vi "getInstanceMsg.vi"(8 "error in (no error)":errorcluster, 11 "tcpServer in":refnum<class "TcpServer.lvclass">) -> (0 "error out":errorcluster, 1 "MsgWrite":refnum<user-event>, 2 "MsgRead":refnum<user-event>, 3 "tcpServer out":refnum<class "TcpServer.lvclass">)   [LabVIEW 2018, in "TcpServer.lvclass"]
doc: "Get the message user event instance.\n\nMsgRead => receive a message from TCP Client.\nMsgWrite => send a message to TCP Client."
uses:
  TcpServer.lvclass
  typedef/eventTypeDef.ctl
  typedef/tcpPacketTypeDef.ctl
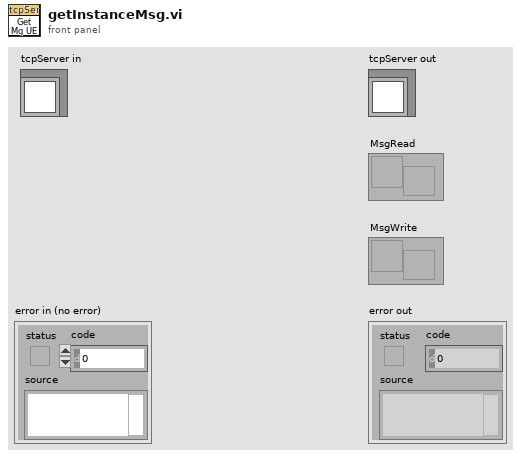
[diagram p1: front panel]
types:
  T1 = typedef "TcpServer.lvclass/userEventTypeDef.ctl" = cluster{"TcpServer":refnum<user-event>, "CmdRead":refnum<user-event>, "CmdWrite":refnum<user-event>, "MsgRead":refnum<user-event>, "MsgWrite":refnum<user-event>, "GenRead":refnum<user-event>, "GenWrite":refnum<user-event>}
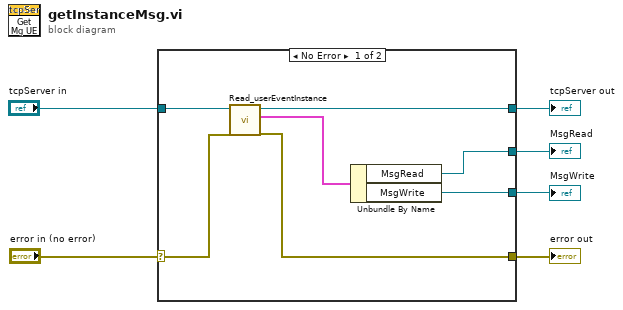
[diagram p0: block diagram]
diagram:
  n1 = case shown="No Error" "error in (no error)" {
    selector: "error in (no error)" -> [w9 w15]
    tunnel: [w8 w15] -> w5
    tunnel: [w12 w14] -> w3
    tunnel: "tcpServer in" -> [w13 w14]
    tunnel: [w10 _] -> w1
    tunnel: [w7 _] -> w2
    frame No Error {
      n2 = call "Read_userEventInstance.vi"("error in (no error)"=w9, "tcpServer in"=w13) -> ("error out"=w8:errorcluster, "UserEvents"=w11:T1, "tcpServer out"=w12:refnum<class "TcpServer.lvclass">)  [unwired: 7 in]
      n3 = Unbundle By Name(w11) -> ("MsgRead"=w10:refnum<user-event>, "MsgWrite"=w7:refnum<user-event>)
    }
    frame Error {
    }
  }
  "error out" <- w5
  "tcpServer out" <- w3
  "MsgWrite" <- w2
  "MsgRead" <- w1
